vi "Slope.vi"(1 "direction":bool, 2 "level":dbl format="%.2f", 3 "array":dbl[](array[numeric]) format="%.2f") -> (0 "index":i32)   [LabVIEW 2009]
panel:
  # "pos"
  # "neg"
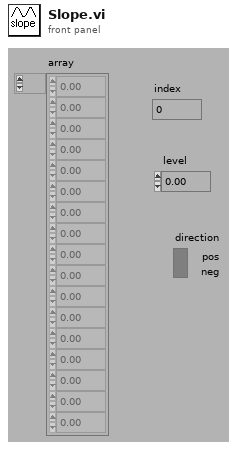
[diagram p1: front panel]
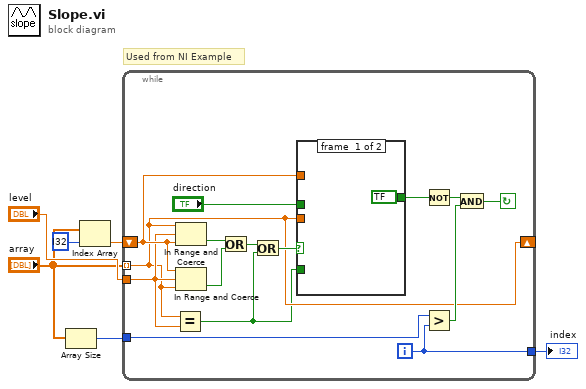
[diagram p0: block diagram]
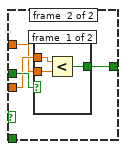
[diagram p2: hidden frame]
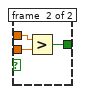
[diagram p3: hidden frame]
diagram:
  # "Used from NI Example"
  n1 = Array Size(array="array") -> (size(s)=w1:i32)
  n2 = Index Array(array="array", index=i32 ?) -> (element=w5:dbl)
  n3 = while {
    tunnel: w1 -> [w16]
    tunnel: [w17] -> w3
    tunnel: "level" -> [w10]
    tunnel: "array" -> [w9] mode=indexing
    shift-left: w5 -> [w18]
    shift-right: [w9] -> _
    i -> [w17]
    stop <- w15 continue-if-true
    n4 = Equal?(x=w9, y=w10) -> (x = y?=w8:bool)
    n5 = In Range and Coerce(upper limit=w9, x=w10, lower limit=w18) -> (In Range?=w19:bool)  [unwired: 1 out]
    n6 = In Range and Coerce(upper limit=w18, x=w10, lower limit=w9) -> (In Range?=w20:bool)  [unwired: 1 out]
    n7 = Or(x=w19, y=w20) -> (x .or. y?=w12:bool)
    n8 = Or(x=w12, y=w8) -> (x .or. y?=w11:bool)
    n9 = case shown="True" w11 {
      tunnel: "direction" -> [_ w26]
      tunnel: w9 -> [_ w25]
      tunnel: w18 -> [_ w24]
      tunnel: w8 -> [_ _]
      tunnel: [bool ? w23] -> w7
      frame #0 {
      }
      frame #1 {
        n10 = case shown="True" w26 {
          tunnel: w25 -> [w29 w32]
          tunnel: w24 -> [w28 w31]
          tunnel: [w27 w30] -> w23
          frame #0 {
            n11 = Less?(x=w29, y=w28) -> (x < y?=w27:bool)
          }
          frame #1 {
            n12 = Greater?(x=w32, y=w31) -> (0:w30:bool)
          }
        }
      }
    }
    n13 = Not(x=w7) -> (.not. x?=w14:bool)
    n14 = Greater?(x=w16, y=w17) -> (0:w13:bool)
    n15 = And(x=w14, y=w13) -> (x .and. y?=w15:bool)
  }
  "index" <- w3
